vi "Get.vi"(8 "error in (no error)":errorcluster, 11 "MsgPackDeserializer in":refnum<class "MsgPackDeserializer.lvclass">) -> (0 "error out":errorcluster, 2 "Variant":variant, 3 "MsgPackDeserializer out":refnum<class "MsgPackDeserializer.lvclass">)   [LabVIEW 2015, in "MsgPackDeserializer.lvclass"]
uses:
  MsgPackDeserializer.lvclass
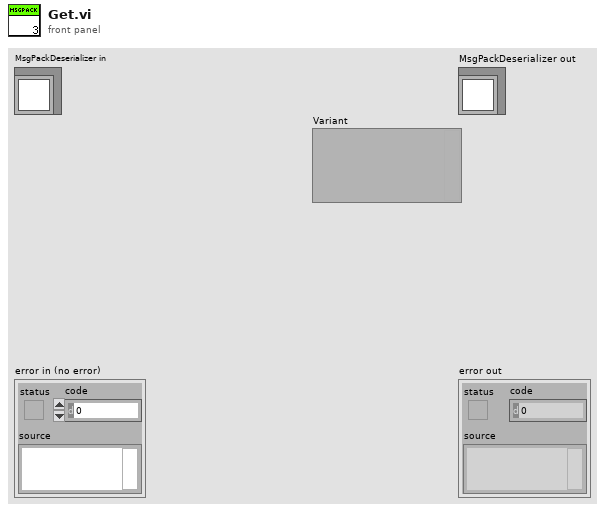
[diagram p1: front panel]
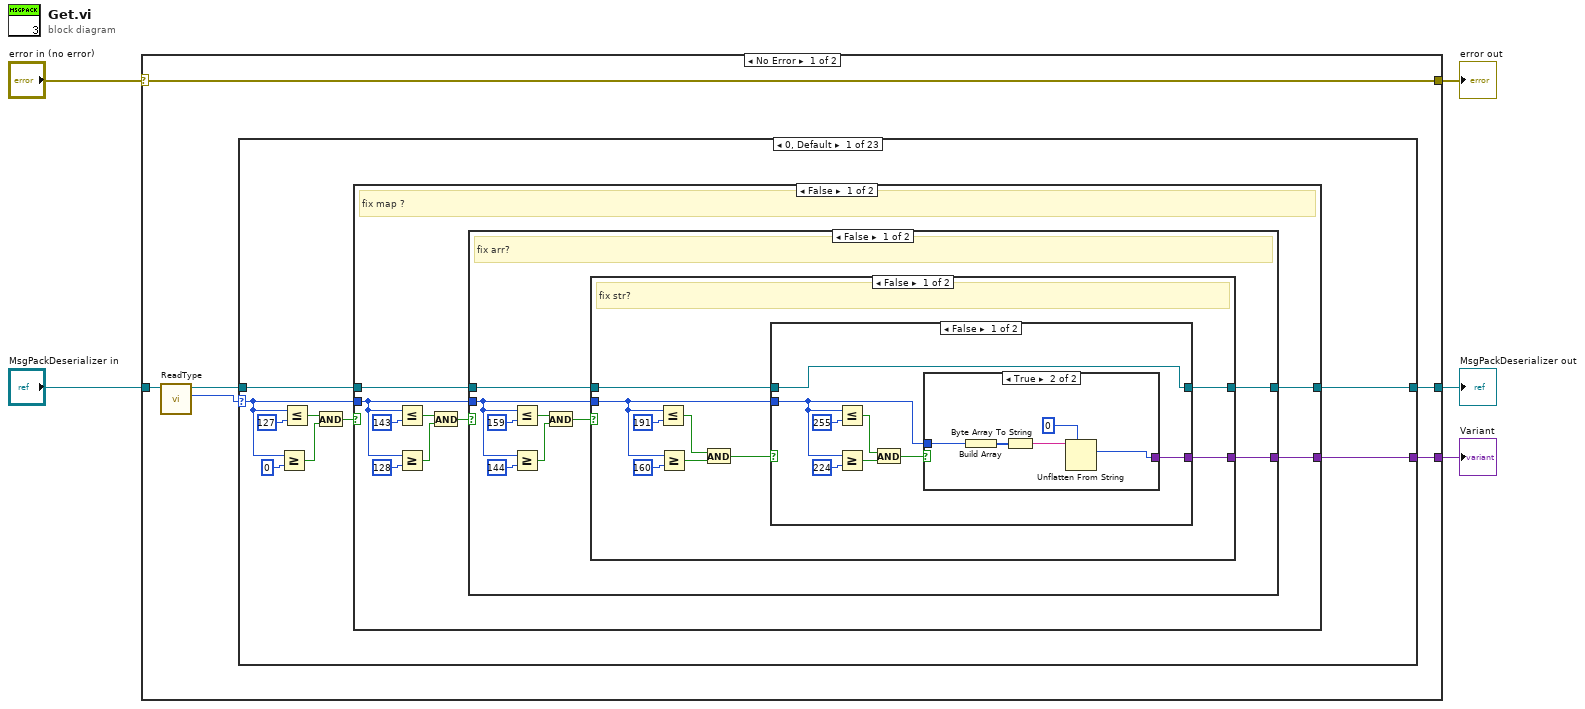
[diagram p0: block diagram]
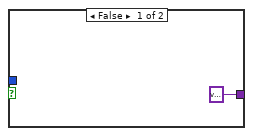
[diagram p2: hidden frame]
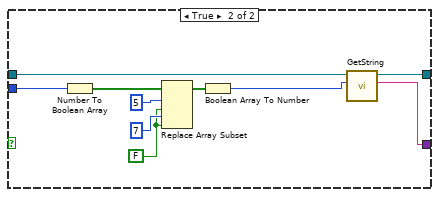
[diagram p3: hidden frame]
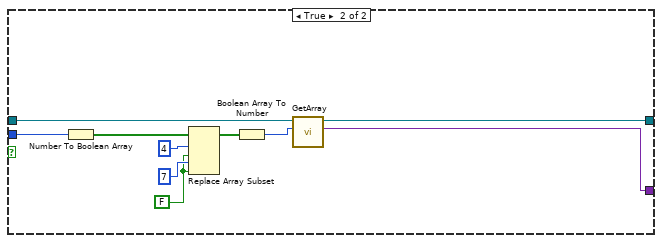
[diagram p4: hidden frame]
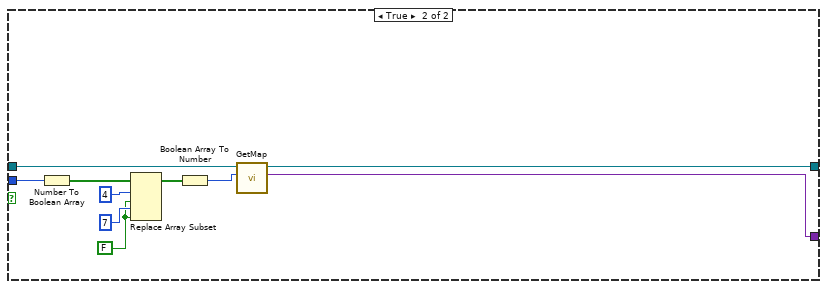
[diagram p5: hidden frame]
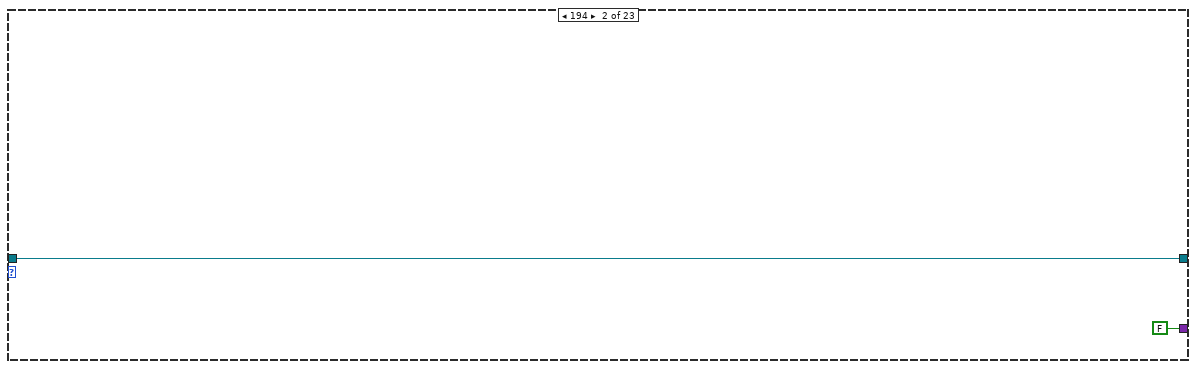
[diagram p7: hidden frame]
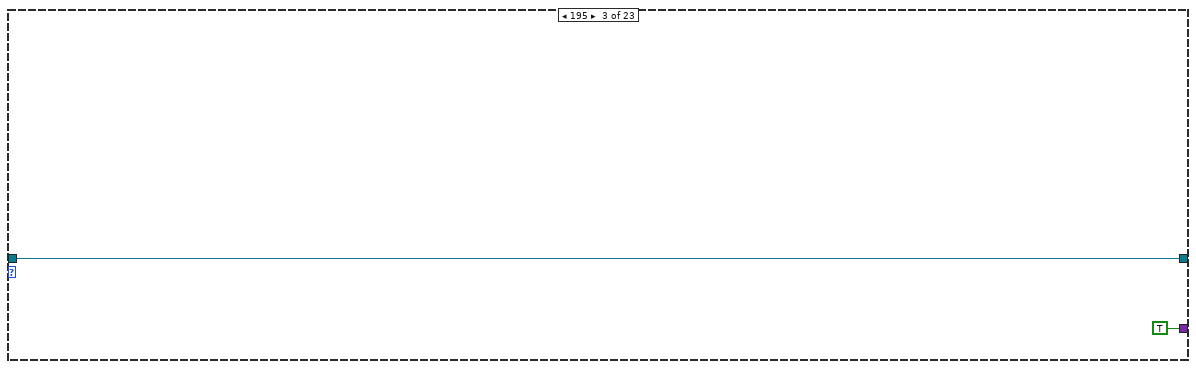
[diagram p8: hidden frame]
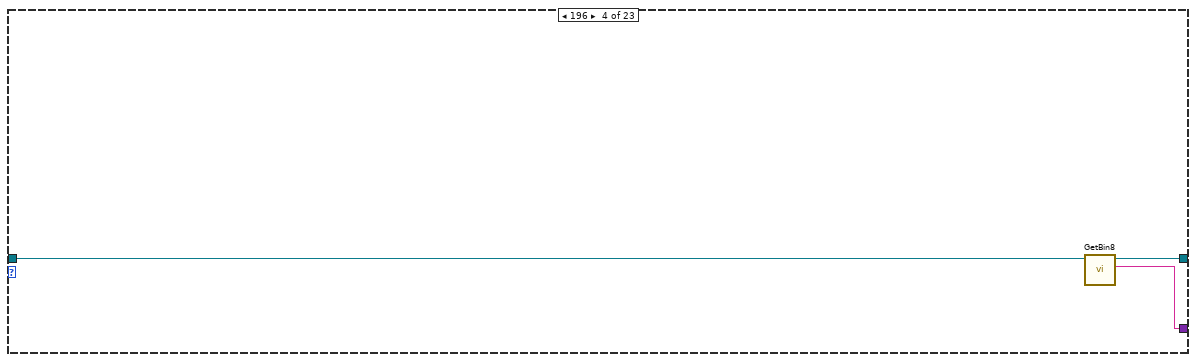
[diagram p9: hidden frame]
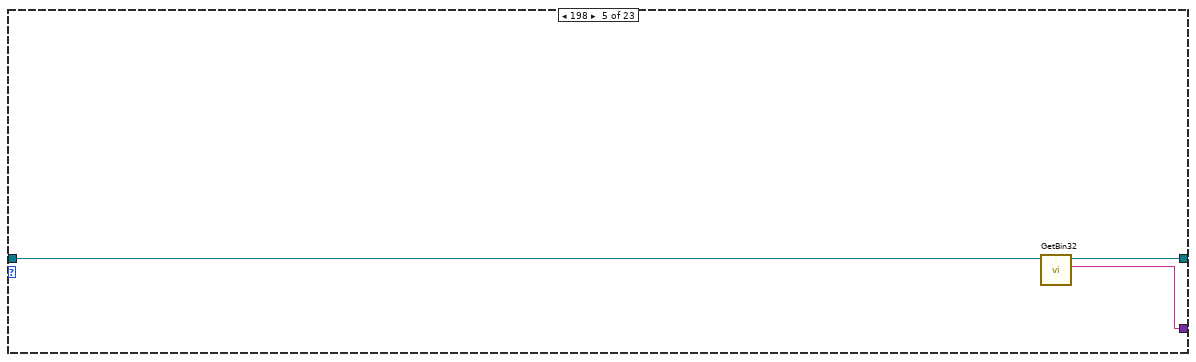
[diagram p10: hidden frame]
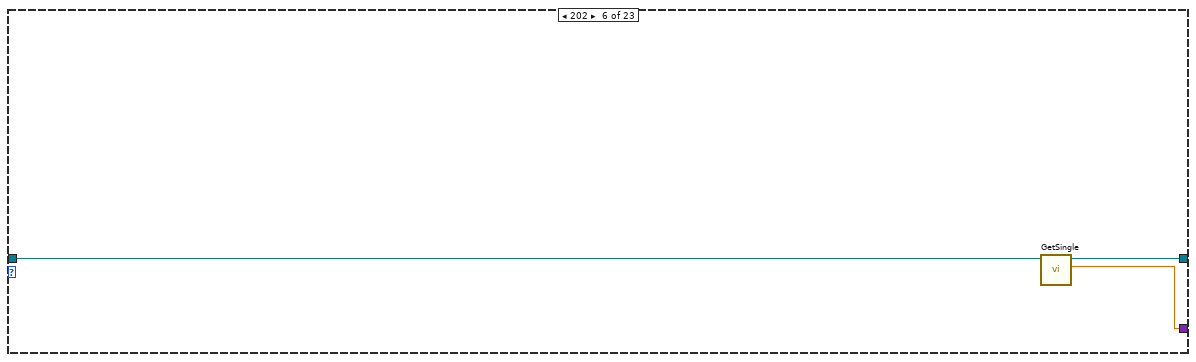
[diagram p11: hidden frame]
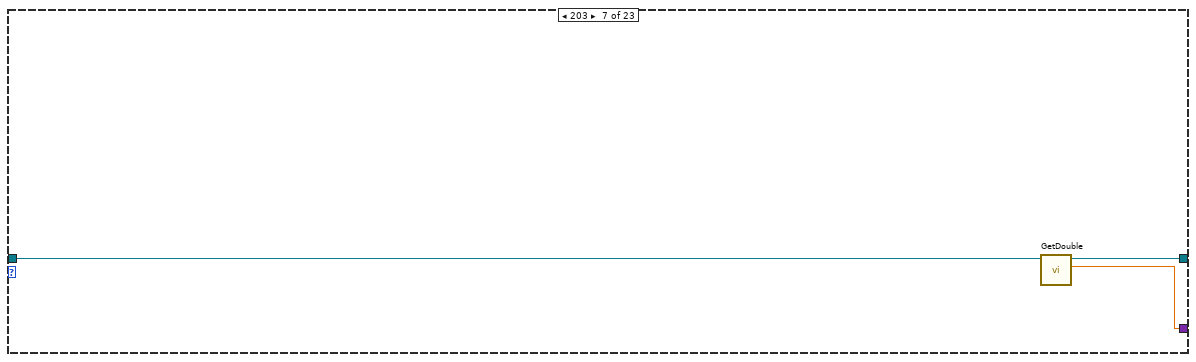
[diagram p12: hidden frame]
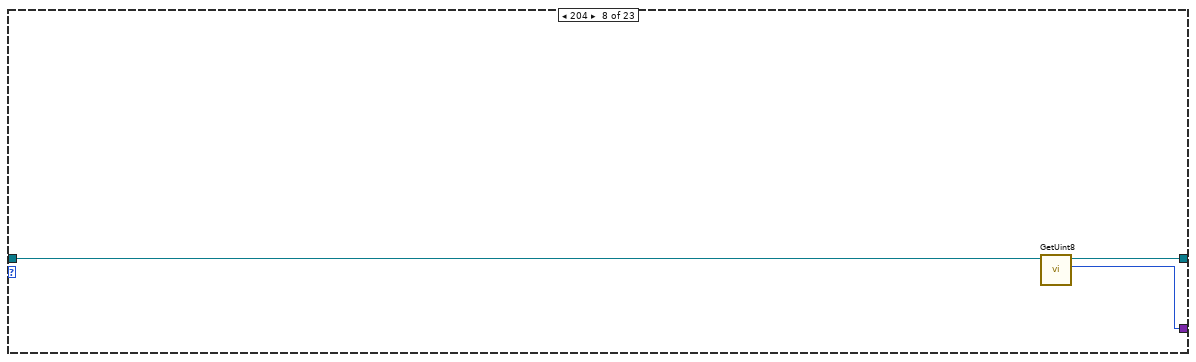
[diagram p13: hidden frame]
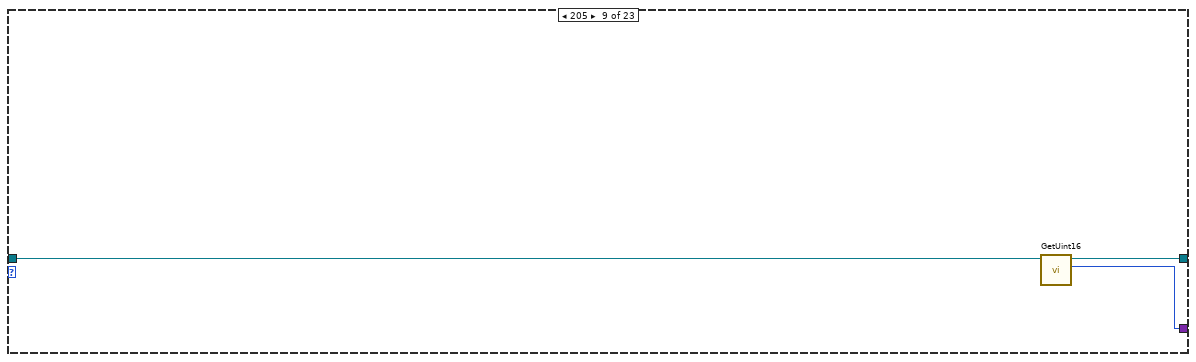
[diagram p14: hidden frame]
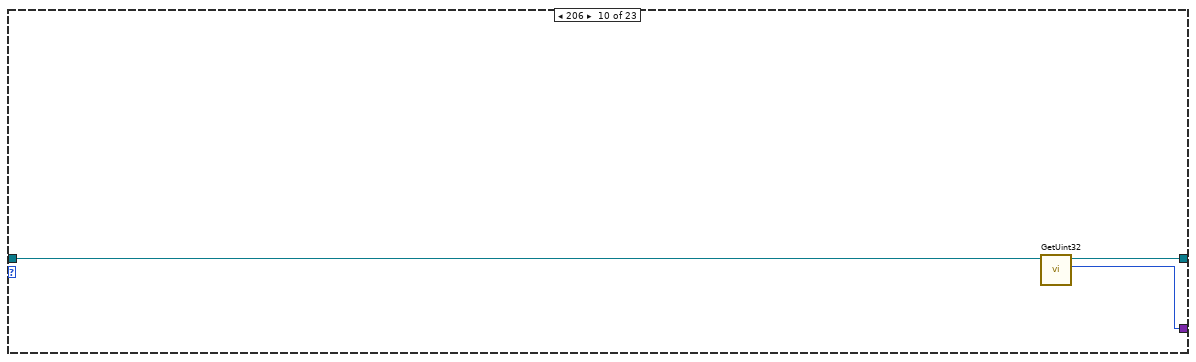
[diagram p15: hidden frame]
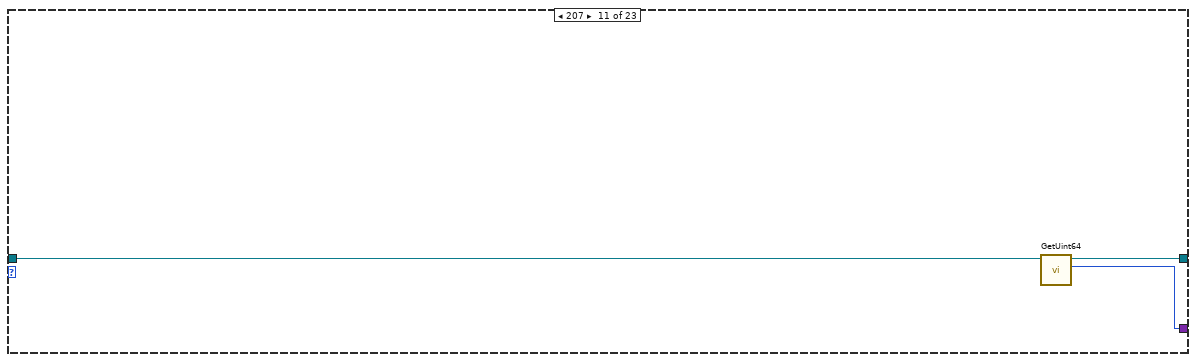
[diagram p16: hidden frame]
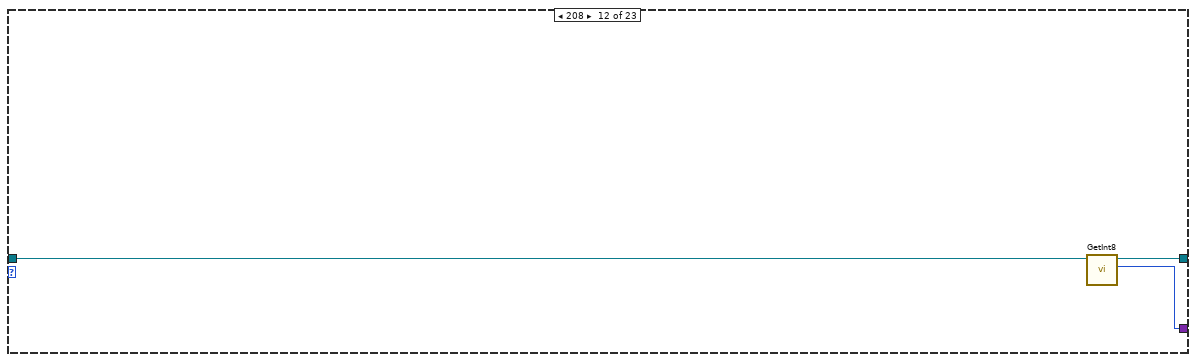
[diagram p17: hidden frame]
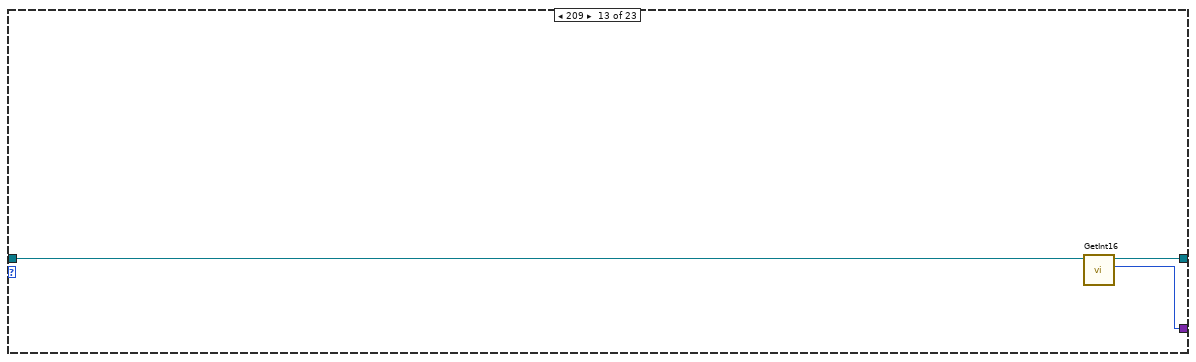
[diagram p18: hidden frame]
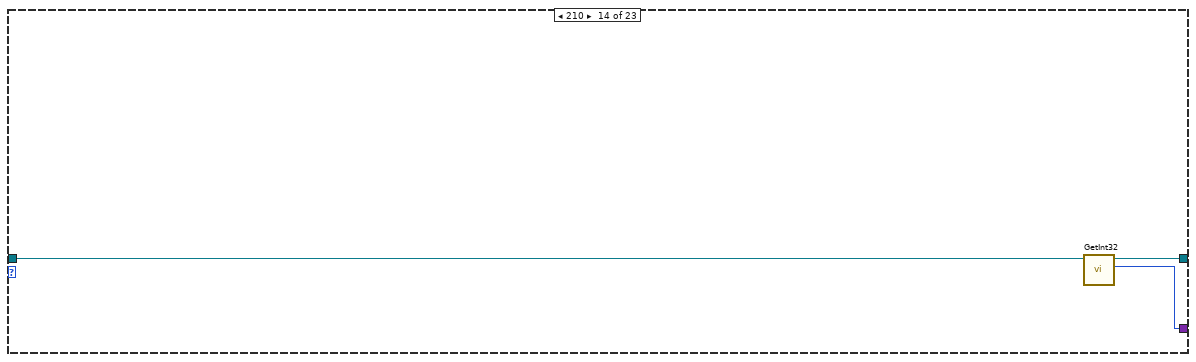
[diagram p19: hidden frame]
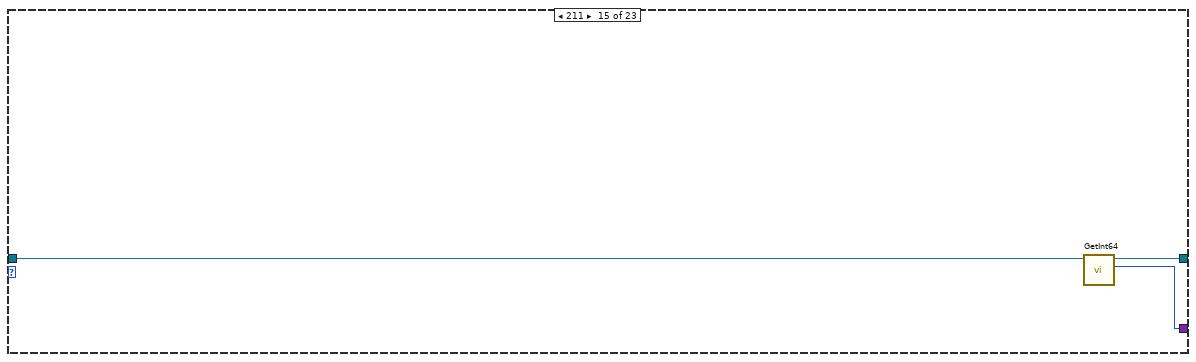
[diagram p20: hidden frame]
diagram:
  n1 = case shown="No Error" "error in (no error)" {
    selector: "error in (no error)" -> [w11 w167]
    tunnel: [w11 w167] -> w4
    tunnel: [w6 w166] -> w2
    tunnel: "MsgPackDeserializer in" -> [w10 w166]
    tunnel: [w8 _] -> w1
    frame No Error {
      n2 = call "ReadType.vi"("MsgPackDeserializer in"=w10) -> ("Type"=w9:u8, "MsgPackDeserializer out"=w7:refnum<class "MsgPackDeserializer.lvclass">)  [unwired: 8 in, 1 out]
      n3 = case shown="0, Default" w9 {
        selector: w9 -> [w13 _ _ _ _ _ _ _ _ _ _ _ _ _ _ _ _ _ _ _ _ _ _]
        tunnel: [w20 FALSE TRUE w100 w101 w104 w107 w110 w113 w117 w119 w123 w126 w129 w132 w134 w138 w141 w144 w152 w153 w158 w164] -> w8
        tunnel: w7 -> [w19 w94 w96 w99 w103 w106 w109 w112 w115 w118 w121 w124 w127 w130 w133 w136 w139 w142 w147 w150 w157 w162 w165]
        tunnel: [w18 w94 w96 w98 w102 w105 w108 w111 w114 w116 w120 w122 w125 w128 w131 w135 w137 w140 w143 w151 w154 w159 w163] -> w6
        frame 0, Default {
          n4 = Greater Or Equal?(x=w13, y=u8 0 ("upper limit")) -> (x >= y?=w17:bool)
          n5 = Less Or Equal?(x=w13, y=u8 127 ("upper limit")) -> (x <= y?=w16:bool)
          n6 = And(x=w16, y=w17) -> (x .and. y?=w14:bool)
          n7 = case shown="False" w14 {
            tunnel: [w29 w93] -> w20
            tunnel: w13 -> [w21 w93]
            tunnel: w19 -> [w28 w92]
            tunnel: [w27 w92] -> w18
            frame False {
              # "fix map ?"
              n8 = Less Or Equal?(x=w21, y=u8 143 ("upper limit")) -> (x <= y?=w25:bool)
              n9 = Greater Or Equal?(x=w21, y=u8 128 ("upper limit")) -> (x >= y?=w26:bool)
              n10 = And(x=w25, y=w26) -> (x .and. y?=w23:bool)
              n11 = case shown="False" w23 {
                tunnel: [w36 w83] -> w29
                tunnel: w21 -> [w30 w86]
                tunnel: w28 -> [w38 w85]
                tunnel: [w37 w84] -> w27
                frame False {
                  # "fix arr?"
                  n12 = Less Or Equal?(x=w30, y=u8 159 ("upper limit")) -> (x <= y?=w35:bool)
                  n13 = Greater Or Equal?(x=w30, y=u8 144 ("upper limit")) -> (x >= y?=w34:bool)
                  n14 = And(x=w35, y=w34) -> (x .and. y?=w33:bool)
                  n15 = case shown="False" w33 {
                    tunnel: w30 -> [w39 w76]
                    tunnel: w38 -> [w47 w75]
                    tunnel: [w46 w72] -> w37
                    tunnel: [w45 w73] -> w36
                    frame False {
                      # "fix str?"
                      n16 = Less Or Equal?(x=w39, y=u8 191 ("upper limit")) -> (x <= y?=w43:bool)
                      n17 = Greater Or Equal?(x=w39, y=u8 160 ("upper limit")) -> (x >= y?=w44:bool)
                      n18 = And(x=w43, y=w44) -> (x .and. y?=w41:bool)
                      n19 = case shown="False" w41 {
                        tunnel: w39 -> [w49 w71]
                        tunnel: w47 -> [w55 w65]
                        tunnel: [w55 w64] -> w46
                        tunnel: [w54 w62] -> w45
                        frame False {
                          n20 = Less Or Equal?(x=w49, y=u8 255 ("upper limit")) -> (x <= y?=w53:bool)
                          n21 = Greater Or Equal?(x=w49, y=u8 224 ("upper limit")) -> (x >= y?=w52:bool)
                          n22 = And(x=w53, y=w52) -> (x .and. y?=w50:bool)
                          n23 = case shown="True" w50 {
                            tunnel: w49 -> [_ w61]
                            tunnel: [variant ("Variant") w57] -> w54
                            frame False {
                            }
                            frame True {
                              n24 = Build Array(w61) -> (w59:u8[])
                              n25 = Byte Array To String(unsigned byte array=w59) -> (string=w60:string)
                              n26 = Unflatten From String(type=i8 0 ("upper limit"), binary string=w60) -> (value=w57:i8)  [unwired: 3 in, 2 out]
                            }
                          }
                        }
                        frame True {
                          w66 = FALSE ("new element/subarray")
                          n27 = Number To Boolean Array(number=w71) -> (Boolean array=w70:bool[])
                          n28 = Replace Array Subset(array=w70, new element #1=w66, index #1=5 ("index"), new element #2=w66, index #2=7 ("index")) -> (w68:bool[])
                          n29 = Boolean Array To Number(Boolean array=w68) -> (number=w63:u32)
                          n30 = call "GetString.vi"("length"=w63, "MsgPackDeserializer in"=w65) -> ("data"=w62:string, "MsgPackDeserializer out"=w64:refnum<class "MsgPackDeserializer.lvclass">)  [unwired: 7 in, 1 out]
                        }
                      }
                    }
                    frame True {
                      w78 = FALSE ("new element/subarray")
                      n31 = Number To Boolean Array(number=w76) -> (Boolean array=w77:bool[])
                      n32 = Replace Array Subset(array=w77, new element #1=w78, index #1=4 ("index"), new element #2=w78, index #2=7 ("index")) -> (w80:bool[])
                      n33 = Boolean Array To Number(Boolean array=w80) -> (number=w74:u32)
                      n34 = call "GetArray.vi"("size"=w74, "MsgPackDeserializer in"=w75) -> ("Variant"=w73:variant, "MsgPackDeserializer out"=w72:refnum<class "MsgPackDeserializer.lvclass">)  [unwired: 7 in, 1 out]
                    }
                  }
                }
                frame True {
                  w88 = FALSE ("new element/subarray")
                  n35 = Number To Boolean Array(number=w86) -> (Boolean array=w87:bool[])
                  n36 = Replace Array Subset(array=w87, new element #1=w88, index #1=4 ("index"), new element #2=w88, index #2=7 ("index")) -> (w90:bool[])
                  n37 = Boolean Array To Number(Boolean array=w90) -> (number=w82:u32)
                  n38 = call "GetMap.vi"("size"=w82, "MsgPackDeserializer in"=w85) -> ("Variant"=w83:variant, "MsgPackDeserializer out"=w84:refnum<class "MsgPackDeserializer.lvclass">)  [unwired: 7 in, 1 out]
                }
              }
            }
            frame True {
              # "fix pos"
            }
          }
        }
        frame 194 {
        }
        frame 195 {
        }
        frame 196 {
          n39 = call "GetBin8.vi"("MsgPackDeserializer in"=w99) -> ("data"=w100:string, "MsgPackDeserializer out"=w98:refnum<class "MsgPackDeserializer.lvclass">)  [unwired: 8 in, 1 out]
        }
        frame 198 {
          n40 = call "GetBin32.vi"("MsgPackDeserializer in"=w103) -> ("data"=w101:string, "MsgPackDeserializer out"=w102:refnum<class "MsgPackDeserializer.lvclass">)  [unwired: 8 in, 1 out]
        }
        frame 202 {
          n41 = call "GetSingle.vi"("MsgPackDeserializer in"=w106) -> ("Number"=w104:sgl, "MsgPackDeserializer out"=w105:refnum<class "MsgPackDeserializer.lvclass">)  [unwired: 8 in, 1 out]
        }
        frame 203 {
          n42 = call "GetDouble.vi"("MsgPackDeserializer in"=w109) -> ("Number"=w107:dbl, "MsgPackDeserializer out"=w108:refnum<class "MsgPackDeserializer.lvclass">)  [unwired: 8 in, 1 out]
        }
        frame 204 {
          n43 = call "GetUint8.vi"("MsgPackDeserializer in"=w112) -> ("Number"=w110:u8, "MsgPackDeserializer out"=w111:refnum<class "MsgPackDeserializer.lvclass">)  [unwired: 8 in, 1 out]
        }
        frame 205 {
          n44 = call "GetUint16.vi"("MsgPackDeserializer in"=w115) -> ("Number"=w113:u16, "MsgPackDeserializer out"=w114:refnum<class "MsgPackDeserializer.lvclass">)  [unwired: 8 in, 1 out]
        }
        frame 206 {
          n45 = call "GetUint32.vi"("MsgPackDeserializer in"=w118) -> ("Number"=w117:u32, "MsgPackDeserializer out"=w116:refnum<class "MsgPackDeserializer.lvclass">)  [unwired: 8 in, 1 out]
        }
        frame 207 {
          n46 = call "GetUint64.vi"("MsgPackDeserializer in"=w121) -> ("Number"=w119:u64, "MsgPackDeserializer out"=w120:refnum<class "MsgPackDeserializer.lvclass">)  [unwired: 8 in, 1 out]
        }
        frame 208 {
          n47 = call "GetInt8.vi"("MsgPackDeserializer in"=w124) -> ("Number"=w123:i8, "MsgPackDeserializer out"=w122:refnum<class "MsgPackDeserializer.lvclass">)  [unwired: 8 in, 1 out]
        }
        frame 209 {
          n48 = call "GetInt16.vi"("MsgPackDeserializer in"=w127) -> ("Number"=w126:i16, "MsgPackDeserializer out"=w125:refnum<class "MsgPackDeserializer.lvclass">)  [unwired: 8 in, 1 out]
        }
        frame 210 {
          n49 = call "GetInt32.vi"("MsgPackDeserializer in"=w130) -> ("Number"=w129:i32, "MsgPackDeserializer out"=w128:refnum<class "MsgPackDeserializer.lvclass">)  [unwired: 8 in, 1 out]
        }
        frame 211 {
          n50 = call "GetInt64.vi"("MsgPackDeserializer in"=w133) -> ("Number"=w132:i64, "MsgPackDeserializer out"=w131:refnum<class "MsgPackDeserializer.lvclass">)  [unwired: 8 in, 1 out]
        }
        frame 217 {
          n51 = call "GetBin8.vi"("MsgPackDeserializer in"=w136) -> ("data"=w134:string, "MsgPackDeserializer out"=w135:refnum<class "MsgPackDeserializer.lvclass">)  [unwired: 8 in, 1 out]
        }
        frame 218 {
          n52 = call "GetBin16.vi"("MsgPackDeserializer in"=w139) -> ("data"=w138:string, "MsgPackDeserializer out"=w137:refnum<class "MsgPackDeserializer.lvclass">)  [unwired: 8 in, 1 out]
        }
        frame 219 {
          n53 = call "GetBin32.vi"("MsgPackDeserializer in"=w142) -> ("data"=w141:string, "MsgPackDeserializer out"=w140:refnum<class "MsgPackDeserializer.lvclass">)  [unwired: 8 in, 1 out]
        }
        frame 220 {
          n54 = call "GetUint16.vi"("MsgPackDeserializer in"=w147) -> ("Number"=w146:u16, "MsgPackDeserializer out"=w145:refnum<class "MsgPackDeserializer.lvclass">)  [unwired: 8 in, 1 out]
          n55 = call "GetArray.vi"("size"=w146, "MsgPackDeserializer in"=w145) -> ("Variant"=w144:variant, "MsgPackDeserializer out"=w143:refnum<class "MsgPackDeserializer.lvclass">)  [unwired: 7 in, 1 out]
        }
        frame 221 {
          n56 = call "GetUint32.vi"("MsgPackDeserializer in"=w150) -> ("Number"=w148:u32, "MsgPackDeserializer out"=w149:refnum<class "MsgPackDeserializer.lvclass">)  [unwired: 8 in, 1 out]
          n57 = call "GetArray.vi"("size"=w148, "MsgPackDeserializer in"=w149) -> ("Variant"=w152:variant, "MsgPackDeserializer out"=w151:refnum<class "MsgPackDeserializer.lvclass">)  [unwired: 7 in, 1 out]
        }
        frame 222 {
          n58 = call "GetUint16.vi"("MsgPackDeserializer in"=w157) -> ("Number"=w156:u16, "MsgPackDeserializer out"=w155:refnum<class "MsgPackDeserializer.lvclass">)  [unwired: 8 in, 1 out]
          n59 = call "GetMap.vi"("size"=w156, "MsgPackDeserializer in"=w155) -> ("Variant"=w153:variant, "MsgPackDeserializer out"=w154:refnum<class "MsgPackDeserializer.lvclass">)  [unwired: 7 in, 1 out]
        }
        frame 223 {
          n60 = call "GetUint32.vi"("MsgPackDeserializer in"=w162) -> ("Number"=w161:u32, "MsgPackDeserializer out"=w160:refnum<class "MsgPackDeserializer.lvclass">)  [unwired: 8 in, 1 out]
          n61 = call "GetMap.vi"("size"=w161, "MsgPackDeserializer in"=w160) -> ("Variant"=w158:variant, "MsgPackDeserializer out"=w159:refnum<class "MsgPackDeserializer.lvclass">)  [unwired: 7 in, 1 out]
        }
        frame 197 {
          n62 = call "GetBin16.vi"("MsgPackDeserializer in"=w165) -> ("data"=w164:string, "MsgPackDeserializer out"=w163:refnum<class "MsgPackDeserializer.lvclass">)  [unwired: 8 in, 1 out]
        }
      }
    }
    frame Error {
    }
  }
  "error out" <- w4
  "MsgPackDeserializer out" <- w2
  "Variant" <- w1
